vi "Datalogging.vi"   [LabVIEW 2019]
uses:
  <vilib>/Rock Robotics/WPI/ThirdParty/Phoenix-LabVIEW/Motor Controller/Get/CTRE_Phoenix_MotorController_GetSelectedSensorData.vi
  Infinite Recharge current/Robot Global Data.vi
  <vilib>/Utility/file.llb/Write Delimited Spreadsheet (string).vi
types:
  T1 = typedef "WPI_MotorControlDeviceRef.ctl" = cluster{"DeviceStatus":errorcluster, "Type":T2, "PWM":cluster{"PWM Channel":T3, "DeadBand":T4}, "CAN":cluster{"Device Number":u8, "SetOutput VI Ref":variant, "GetOutput VI Ref":variant, "Enable VI Ref":variant, "Disable VI Ref":variant, "Data":variant}, "Invert":bool, "DIO PWM":cluster{"PWM \"Enable\" Channel":T3, "DIOChannel":T5, "PWM Rate":dbl}}
  T2 = typedef "WPI_MotorControlType.ctl" = enum16{"PWM", "CAN", "DIO PWM"}
  T3 = typedef "FPGA_DIOPWMChannel.ctl" = enum8{"PWM 0", "PWM 1", "PWM 2", "PWM 3", "PWM 4", "PWM 5", "PWM 6", "PWM 7", "PWM 8", "PWM 9", "PWM MXP 0", "PWM MXP 1", "PWM MXP 2", "PWM MXP 3", "PWM MXP 4", "PWM MXP 5", "PWM MXP 6", "PWM MXP 7", "PWM MXP 8", "PWM MXP 9", "Invalid"}
  T4 = typedef "WPI_PWMDeadband.ctl" = cluster{"Name":string, "maxPositivePwm":i32, "minPositivePwm":i32, "centerPwm":i32, "maxNegativePwm":i32, "minNegativePwm":i32, "angularRange":u16}
  T5 = typedef "FPGA_DIOChannel.ctl" = enum8{"DIO 0", "DIO 1", "DIO 2", "DIO 3", "DIO 4", "DIO 5", "DIO 6", "DIO 7", "DIO 8", "DIO 9", "DIO MXP 0", "DIO MXP 1", "DIO MXP 2", "DIO MXP 3", "DIO MXP 4", "DIO MXP 5", "DIO MXP 6", "DIO MXP 7", "DIO MXP 8", "DIO MXP 9", "DIO MXP 10", "DIO MXP 11", "DIO MXP 12", "DIO MXP 13", "DIO MXP 14", "DIO MXP 15", "SPI Port CS1", "SPI Port CS2", "SPI Port CS3", "SPI Port MISO", "SPI Port MOSI", "Invalid"}
  T6 = cluster{"Yaw":dbl, "Roll":dbl, "Pitch":dbl, "Heading":dbl, "Fused Heading":dbl}
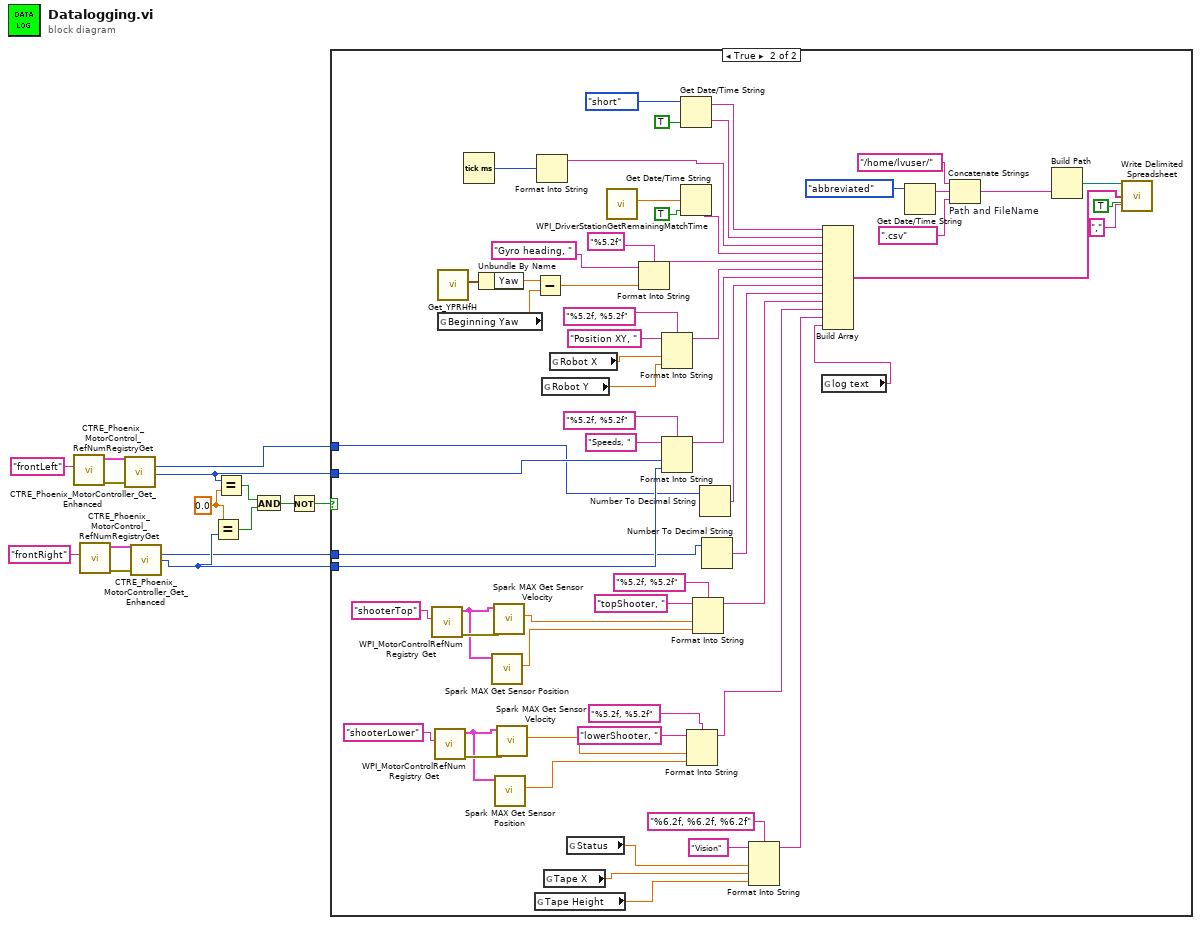
[diagram p0: block diagram]
diagram:
  w15 = 0.0 ("y")
  n1 = call <vilib>:"CTRE_Phoenix_MotorControl_RefNumRegistryGet.vi"("refnum name"="frontLeft") -> ("error out"=w10:errorcluster, "PhoenixMotorControlDevRef"=w9:T1)  [unwired: 9 in]
  n2 = call <vilib>:"CTRE_Phoenix_MotorControl_RefNumRegistryGet.vi"("refnum name"="frontRight") -> ("error out"=w6:errorcluster, "PhoenixMotorControlDevRef"=w5:T1)  [unwired: 9 in]
  n3 = call-poly <vilib>:"CTRE_Phoenix_MotorController_Get_Enhanced.vi"("PhoenixMotorControlDevRef"=w9, "error in"=w10) -> ("Position (Raw Sensor Units)"=w2:i32, "Velocity (Raw Sensor Units per 100 ms)"=w7:i32)  [unwired: 10 in, 2 out]
  n4 = call-poly <vilib>:"CTRE_Phoenix_MotorController_Get_Enhanced.vi"("PhoenixMotorControlDevRef"=w5, "error in"=w6) -> ("Position (Raw Sensor Units)"=w1:i32, "Velocity (Raw Sensor Units per 100 ms)"=w3:i32)  [unwired: 10 in, 2 out]
  n5 = Equal?(x=w15, y=w3) -> (x = y?=w13:bool)
  n6 = Equal?(x=w7, y=w15) -> (x = y?=w14:bool)
  n7 = And(x=w14, y=w13) -> (x .and. y?=w12:bool)
  n8 = Not(x=w12) -> (.not. x?=w11:bool)
  n9 = case shown="True" w11 {
    tunnel: w7 -> [_ w50]
    tunnel: w3 -> [_ w49]
    tunnel: w2 -> [_ w48]
    tunnel: w1 -> [_ w47]
    frame False {
    }
    frame True {
      n10 = call <vilib>:"WPI_MotorControlRefNum Registry Get.vi"("refnum name"="shooterTop") -> ("error out"=w41:errorcluster, "MotorControlDevRef"=w20:T1)  [unwired: 9 in]
      n11 = call <vilib>:"WPI_MotorControlRefNum Registry Get.vi"("refnum name"="shooterLower") -> ("error out"=w29:errorcluster, "MotorControlDevRef"=w19:T1)  [unwired: 9 in]
      n12 = call <vilib>:"Get_YPRHfH.vi"() -> ("YRPHfH"=w16:T6)  [unwired: 11 in]
      n13 = global read "Robot Global Data.vi" "Beginning Yaw"() -> (w18:dbl)
      n14 = Tick Count (ms)() -> (millisecond timer value=w52:u32)
      n15 = Unbundle By Name(w16) -> ("Yaw"=w17:dbl)
      n16 = call <vilib>:"Spark MAX Get Sensor Position.vi"("MotorControlDevRef in"=w20) -> ("Sensor Position"=w30:dbl)  [unwired: 7 in, 3 out]
      n17 = call <vilib>:"Spark MAX Get Sensor Velocity.vi"("error in (no error)"=w41, "MotorControlDevRef in"=w20) -> ("Sensor Velocity"=w31:dbl)  [unwired: 6 in, 3 out]
      n18 = call <vilib>:"Spark MAX Get Sensor Position.vi"("MotorControlDevRef in"=w19) -> ("Sensor Position"=w25:dbl)  [unwired: 7 in, 3 out]
      n19 = call <vilib>:"Spark MAX Get Sensor Velocity.vi"("error in (no error)"=w29, "MotorControlDevRef in"=w19) -> ("Sensor Velocity"=w26:dbl)  [unwired: 6 in, 3 out]
      n20 = Subtract(x=w17, y=w18) -> (x-y=w71:dbl)
      n21 = global read "Robot Global Data.vi" "Tape Height"() -> (w37:dbl)
      n22 = Format Into String(w52) -> (resulting string=w51:string)  [unwired: 3 in, 1 out]
      n23 = global read "Robot Global Data.vi" "Robot Y"() -> (w34:dbl)
      n24 = global read "Robot Global Data.vi" "Tape X"() -> (w36:dbl)
      n25 = global read "Robot Global Data.vi" "Robot X"() -> (w35:dbl)
      n26 = global read "Robot Global Data.vi" "Status"() -> (w38:dbl)
      n27 = call <vilib>:"WPI_DriverStationGetRemainingMatchTime.vi"() -> ("Match Time(s)"=w77:sgl)  [unwired: 10 in, 1 out]
      n28 = Format Into String(format string="%5.2f", initial string="Gyro heading, " ("element"), w71) -> (resulting string=w55:string)  [unwired: 1 in, 1 out]
      n29 = Format Into String(format string="%5.2f, %5.2f", initial string="Position XY, ", w35, w34) -> (resulting string=w54:string)  [unwired: 1 in, 1 out]
      n30 = Format Into String(format string="%5.2f, %5.2f", initial string="Speeds, ", w50, w49) -> (resulting string=w53:string)  [unwired: 1 in, 1 out]
      n31 = Get Date/Time String(date format (0)=enum16{"short", "long", "abbreviated"}."short", want seconds? (F)=TRUE) -> (date string=w64:string, time string=w63:string)  [unwired: 1 in]
      n32 = Get Date/Time String(seconds (now)=w77, want seconds? (F)=TRUE) -> (time string=w73:string)  [unwired: 1 in, 1 out]
      n33 = Format Into String(format string="%5.2f, %5.2f", initial string="lowerShooter, ", w26, w25) -> (resulting string=w24:string)  [unwired: 1 in, 1 out]
      n34 = Format Into String(format string="%5.2f, %5.2f", initial string="topShooter, ", w31, w30) -> (resulting string=w22:string)  [unwired: 1 in, 1 out]
      n35 = Number To Decimal String(number=w48) -> (decimal integer string=w46:string)  [unwired: 1 in]
      n36 = Number To Decimal String(number=w47) -> (decimal integer string=w45:string)  [unwired: 1 in]
      n37 = Format Into String(format string="%6.2f, %6.2f, %6.2f", initial string="Vision", w38, w36, w37) -> (resulting string=w42:string)  [unwired: 1 in, 1 out]
      n38 = global read "Robot Global Data.vi" "log text"() -> (w33:string)
      n39 = Build Array(w64, w63, w51, w73, w55, w54, w53, w46, w45, w22, w24, w42, w33) -> (w39:string[])
      n40 = Get Date/Time String(date format (0)=enum16{"short", "long", "abbreviated"}."abbreviated") -> (date string=w65:string)  [unwired: 2 in, 1 out]
      n41 = Concatenate Strings "Path and FileName"("/home/lvuser/", w65, ".csv") -> (w68:string)
      n42 = Build Path(name or relative path=w68) -> (appended path=w67:path)  [unwired: 1 in]
      n43 = call-poly <vilib>:"Write Delimited Spreadsheet.vi"("file path (dialog if empty)"=w67, "1D data"=w39, "append to file? (new file:F)"=TRUE, "delimiter (\\t)"="," ("delimiter (\\t)")) -> ()  [unwired: 10 in, 2 out]
    }
  }
